vi "WriteResponse.vi"(8 "error in (no error)":errorcluster, 9 "Value":u16 format="%x", 11 "connection ID In":refnum<k5>) -> (0 "error out":errorcluster, 3 "connection ID out":refnum<k5>)   [LabVIEW 2017]
uses:
  Controls/FrameHeader.ctl
  Controls/RegisterAddress.ctl
panel:
  in  "Register":T1 items=["Mode0"=1, "Status"=3, "ImageDataFormat"=4, "IntegrationTime"=5, "DeviceType"=6, "Deviceinfo"=7, "Firmwareinfo"=8, "ModulationFrequency"=9, "FramRate"=10, ""=0]
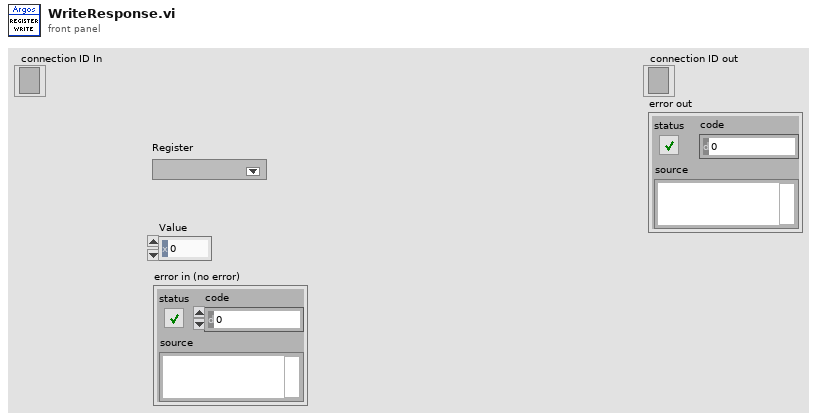
[diagram p1: front panel]
types:
  T1 = typedef "RegisterAddress.ctl" = u16
  T2 = typedef "FrameHeader.ctl" = cluster{"Protocol Version (8)":u8, "Command (8)":u8, "SubCommand (8)":u8, "Status (8)":u8, "Length (32)":u32, "Register Address (32)":u16, "HeaderData2 (8)":u8, "Flags (16)":u16, "HeaderData3 (8)":u8}
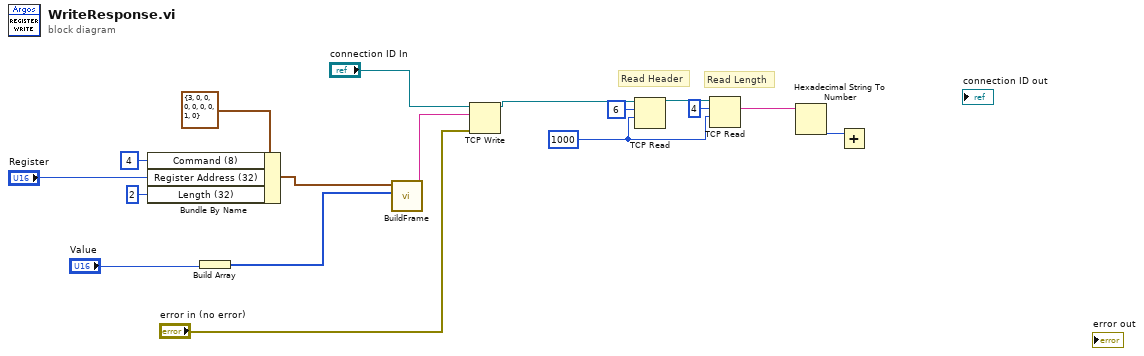
[diagram p0: block diagram]
diagram:
  w3 = 1000 ("timeout ms (25000)")
  # "Read Length"
  # "Read Header"
  n1 = Bundle By Name(cluster=T2 {"Protocol Version (8)"=3, "Command (8)"=0, "SubCommand (8)"=0, "Status (8)"=0, "Length (32)"=0, "Register Address (32)"=0, "HeaderData2 (8)"=0, "Flags (16)"=1, "HeaderData3 (8)"=0} ("Header"), "Command (8)"=u8 4, "Register Address (32)"="Register", "Length (32)"=u32 2) -> (w14:T2)
  n2 = Build Array("Value") -> (w13:u16[])
  n3 = call "BuildFrame.vi"("Data"=w13, "Header"=w14) -> ("FrameOut"=w12:string)  [unwired: 9 in]
  n4 = TCP Write(connection ID="connection ID In", data in=w12, error in (no error)="error in (no error)") -> (connection ID out=w7:refnum<k5>)  [unwired: 1 in, 2 out]
  n5 = TCP Read(connection ID=w7, bytes to read=u16 6, 9:w3) -> (connection ID out=w5:refnum<k5>)  [unwired: 2 in, 2 out]
  n6 = TCP Read(connection ID=w5, bytes to read=4, 9:w3) -> (data out=w2:string)  [unwired: 2 in, 2 out]
  n7 = Hexadecimal String To Number(string=w2) -> (number=w1:u32)  [unwired: 2 in, 1 out]
  n8 = Add(x=w1) -> ()  [unwired: 1 in, 1 out]
